vi "DAQ_Setup.vi"(11 "Params":T1={"Sample Clock Source"="OnboardClock", "Sample Rate"=48000, "Hammer"={"Physical Channel"="Dev2/ai0", "Terminal Configuration"=12529, "IEPE Source"=10200, "Current (A)"=0.004, "Trigger"=0, "Min Force"=-100.0, "Max Force"=100.0, "Force Sensitivity (mV/N)"=50.0}, "Microphone"={"Physical Channel"="Dev2/ai1", "Terminal Configuration"=12529, "IEPE Source"=10200, "Current (A)"=0.004, "Output"=2, "Min SPL/Acc"=0.0, "Max SPL/Acc"=120.0, "Sensitivity (mV/g or mV/Pa)"=10.0}} {"Microphone"."Output" items=["Accelerometer", "Accel (speed)", "Microphone", "Vibrometer"]; "Microphone"."IEPE Source" items=["Internal"=10200, "External"=10167, "None"=10230]; "Microphone"."Terminal Configuration" items=["default"=-1, "RSE"=10083, "NRSE"=10078, "Differential"=10106, "Pseudodifferential"=12529]; "Hammer"."Trigger" items=["Hammer (force)", "Self-tap"]; "Hammer"."IEPE Source" items=["Internal"=10200, "External"=10167, "None"=10230]; "Hammer"."Terminal Configuration" items=["default"=-1, "RSE"=10083, "NRSE"=10078, "Differential"=10106, "Pseudodifferential"=12529]}) -> (0 "error out":errorcluster, 1 "SampClk.Rate":dbl, 2 "Y axis Label":string, 3 "Task out":refnum<k21>, 4 "Sensitivity (mV/X)":dbl[](array[numeric]))   [LabVIEW 2021]
uses:
  <vilib>/DAQmx/create/channels.llb/DAQmx Create Channel (AI-Acceleration-Accelerometer).vi
  <vilib>/DAQmx/create/channels.llb/DAQmx Create Channel (AI-Force-IEPE Sensor).vi
  <vilib>/DAQmx/create/channels.llb/DAQmx Create Channel (AI-Sound Pressure-Microphone).vi
  <resource>/objmgr/daqmx.rc
  <vilib>/DAQmx/configure/timing.llb/DAQmx Timing (Sample Clock).vi
panel:
  # "Timing Settings"
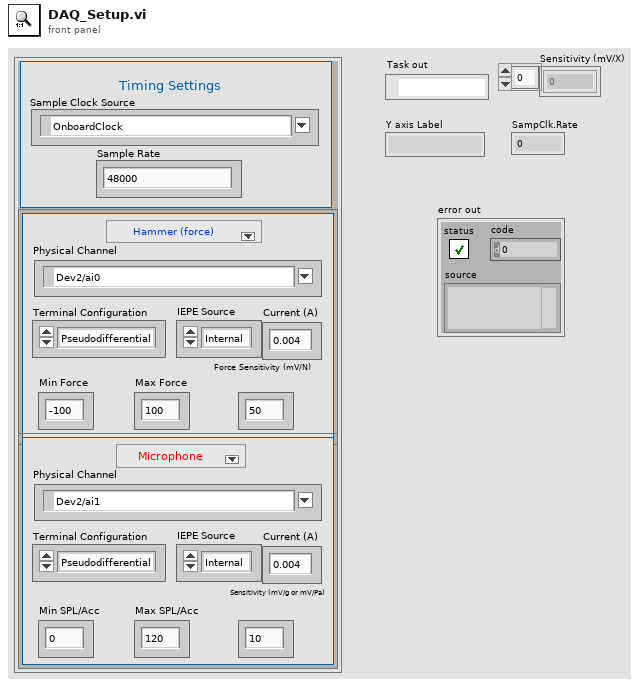
[diagram p1: front panel]
types:
  T1 = cluster{"Sample Clock Source":tag, "Sample Rate":u32, "Hammer":cluster{"Physical Channel":tag, "Terminal Configuration":i32, "IEPE Source":i32, "Current (A)":dbl, "Trigger":u16, "Min Force":dbl, "Max Force":dbl, "Force Sensitivity (mV/N)":dbl}, "Microphone":cluster{"Physical Channel":tag, "Terminal Configuration":i32, "IEPE Source":i32, "Current (A)":dbl, "Output":u16, "Min SPL/Acc":dbl, "Max SPL/Acc":dbl, "Sensitivity (mV/g or mV/Pa)":dbl}}
  T2 = enum32{"Acceleration", "Sound Pressure", "Force"}[][]
  T3 = cluster{"Physical Channel":tag, "Terminal Configuration":i32, "IEPE Source":i32, "Current (A)":dbl, "Trigger":u16, "Min Force":dbl, "Max Force":dbl, "Force Sensitivity (mV/N)":dbl}
  T4 = cluster{"Physical Channel":tag, "Terminal Configuration":i32, "IEPE Source":i32, "Current (A)":dbl, "Output":u16, "Min SPL/Acc":dbl, "Max SPL/Acc":dbl, "Sensitivity (mV/g or mV/Pa)":dbl}
  T5 = cluster{"Hammer":cluster{"Physical Channel":tag, "Terminal Configuration":i32, "IEPE Source":i32, "Current (A)":dbl, "Trigger":u16, "Min Force":dbl, "Max Force":dbl, "Force Sensitivity (mV/N)":dbl}, "Microphone":cluster{"Physical Channel":tag, "Terminal Configuration":i32, "IEPE Source":i32, "Current (A)":dbl, "Output":u16, "Min SPL/Acc":dbl, "Max SPL/Acc":dbl, "Sensitivity (mV/g or mV/Pa)":dbl}}
  T6 = cluster{"Physical Channel":tag, "Terminal Configuration":i32, "IEPE Source":i32, "Current (A)":dbl, "Output":u16, "Min SPL/Acc":dbl, "Max SPL/Acc":dbl, "Sensitivity (mV/g or mV/Pa)":dbl}[]
  T7 = enum32{"Acceleration", "Sound Pressure", "Force"}
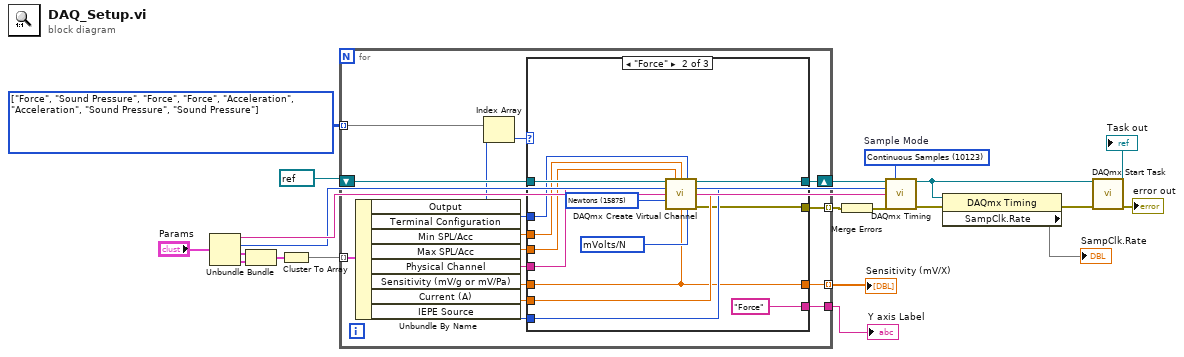
[diagram p0: block diagram]
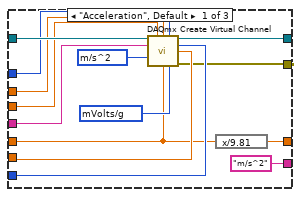
[diagram p2: hidden frame]
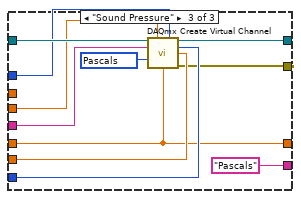
[diagram p3: hidden frame]
diagram:
  w11 = 10123 items=["Finite Samples"=10178, "Continuous Samples"=10123, "Hardware Timed Single Point"=12522]  # Sample Mode
  w20 = T2 [[enum."Force", enum."Sound Pressure", enum."Force", enum."Force"], [enum."Acceleration", enum."Acceleration", enum."Sound Pressure", enum."Sound Pressure"]] items=["Acceleration", "Sound Pressure", "Force"]
  n1 = Unbundle("Params") -> ("Sample Clock Source"=w4:tag, "Sample Rate"=w3:u32, "Hammer"=w15:T3, "Microphone"=w14:T4)
  n2 = Bundle("Hammer"=w15, "Microphone"=w14) -> (w13:T5)  [unwired: 1 in]
  n3 = Cluster To Array(cluster=w13) -> (array=w19:T6)
  n4 = for {
    tunnel: [w36] -> w16 mode=indexing
    tunnel: [w35] -> w21
    shift-right: [w37] -> w7
    shift-left: refnum<k21> refnum ("task in") -> [w31]
    tunnel: w19 -> [w30] mode=indexing
    tunnel: w20 -> [w29] mode=indexing
    tunnel: [w22] -> w1 mode=indexing
    n5 = Unbundle By Name(w30) -> ("Output"=w27:u16, "Terminal Configuration"=w24:i32, "Min SPL/Acc"=w25:dbl, "Max SPL/Acc"=w26:dbl, "Physical Channel"=w34:tag, "Sensitivity (mV/g or mV/Pa)"=w28:dbl, "Current (A)"=w33:dbl, "IEPE Source"=w32:i32)
    n6 = Index Array(array=w29, index=w27) -> (element=w23:T7)
    n7 = case shown="\"Force\"" w23 {
      tunnel: [w44 w54 w69] -> w36
      tunnel: [w51 w64 w75] -> w37
      tunnel: w34 -> [w43 w58 w66]
      tunnel: w32 -> [w45 w60 w71]
      tunnel: w33 -> [w46 w59 w70]
      tunnel: ["m/s^2" ("RingText.Text") "Force" ("RingText.Text") "Pascals" ("RingText.Text")] -> w35
      tunnel: w31 -> [w47 w63 w72]
      tunnel: w28 -> [w39 w52 w65]
      tunnel: w26 -> [w42 w57 w68]
      tunnel: w25 -> [w41 w56 _]
      tunnel: w24 -> [w40 w55 w67]
      tunnel: [w38 w52 w65] -> w22
      frame "Acceleration", Default {
        w50 = 12509 items=["mVolts/g"=12509, "Volts/g"=12510] ("Sensitivity Units")
        w49 = 12470 items=["g"=10186, "m/s^2"=12470, "in/s^2"=12471, "From Custom Scale"=10065] ("Acceleration Units")
        n8 = call-poly <vilib>:"DAQmx Create Virtual Channel.vi"("task in"=w47, "maximum value"=w42, "minimum value"=w41, "input terminal configuration"=w40, "physical channels"=w43, "current excitation source"=w45, "current excitation value"=w46, "units"=w49, "sensitivity"=w39, "sensitivity units"=w50) -> ("task out"=w51:refnum<k21>, "error out"=w44:errorcluster)  [unwired: 4 in]
        n9 = expression code="x/9.81"(w39) -> (w38:dbl)
      }
      frame "Force" {
        w62 = 15875 items=["Newtons"=15875, "Pounds"=15876, "From Custom Scale"=10065] ("Force Units")
        w61 = 15891 items=["mVolts/N"=15891, "mVolts/lb"=15892] ("Force Sensitivity Units")
        n10 = call-poly <vilib>:"DAQmx Create Virtual Channel.vi"("task in"=w63, "maximum value"=w57, "minimum value"=w56, "input terminal configuration"=w55, "physical channels"=w58, "current excitation source"=w60, "current excitation value"=w59, "units"=w62, "sensitivity"=w52, "sensitivity units"=w61) -> ("task out"=w64:refnum<k21>, "error out"=w54:errorcluster)  [unwired: 4 in]
      }
      frame "Sound Pressure" {
        w73 = 10081 items=["Pascals"=10081, "From Custom Scale"=10065] ("Sound Pressure Units")
        n11 = call-poly <vilib>:"DAQmx Create Virtual Channel.vi"("task in"=w72, "maximum sound pressure level"=w68, "input terminal configuration"=w67, "physical channels"=w66, "current excitation source"=w71, "current excitation value"=w70, "units"=w73, "microphone sensitivity"=w65) -> ("task out"=w75:refnum<k21>, "error out"=w69:errorcluster)  [unwired: 6 in]
      }
    }
  }
  "Y axis Label" <- w21
  "Sensitivity (mV/X)" <- w1
  n12 = Merge Errors(w16) -> (w6:errorcluster)
  n13 = call-poly <vilib>:"DAQmx Timing.vi"("task/channels in"=w7, "sample mode"=w11, "rate"=w3, "source"=w4, "error in"=w6) -> ("task out"=w9:refnum<k21>, "error out"=w12:errorcluster)  [unwired: 9 in]
  n14 = property class="DAQmx Timing"(reference=w9, error in=w12) -> (error out=w10:errorcluster, "SampClk.Rate"=→"SampClk.Rate")  [unwired: 1 out]
  n15 = call <vilib>:"DAQmx Start Task.vi"("task/channels in"=w9, "error in"=w10) -> ("task out"=→"Task out":refnum<k21>, "error out"=→"error out":errorcluster)  [unwired: 12 in]
